vi "Combine Events.vi"(5 "NXT":T1={"Hardware"="NXT", "Flattened String"=""}) -> (1 "4134 Events":u8[](array[numeric]), 2 "NXT":T1={"Hardware"="NXT", "Flattened String"=""})   [LabVIEW 2010, in "FTC.lvlib" / "Remote Interface.lvlib"]
uses:
  Remote Interface.lvlib
  <vilib>/FTC/FTC POVState.ctl
  <vilib>/NXT/Subs/LVHSConnector.ctl
  <vilib>/NXT/Dual Mode Library/prims/dataManipulation/joinU8.vi
panel:
  in  "Old Button Encoding 2":u16
  in  "Old POV 2":T2 items=["None"=-1, "POV Up"=0, "POV Up Right"=1, "POV Right"=2, "POV Down Right"=3, "POV Down"=4, "POV Down Left"=5, "POV Left"=6, "POV Up Left"=7]
  in  "Old Button Encoding 1":u16
  in  "Old POV 1":T2 items=["None"=-1, "POV Up"=0, "POV Up Right"=1, "POV Right"=2, "POV Down Right"=3, "POV Down"=4, "POV Down Left"=5, "POV Left"=6, "POV Up Left"=7]
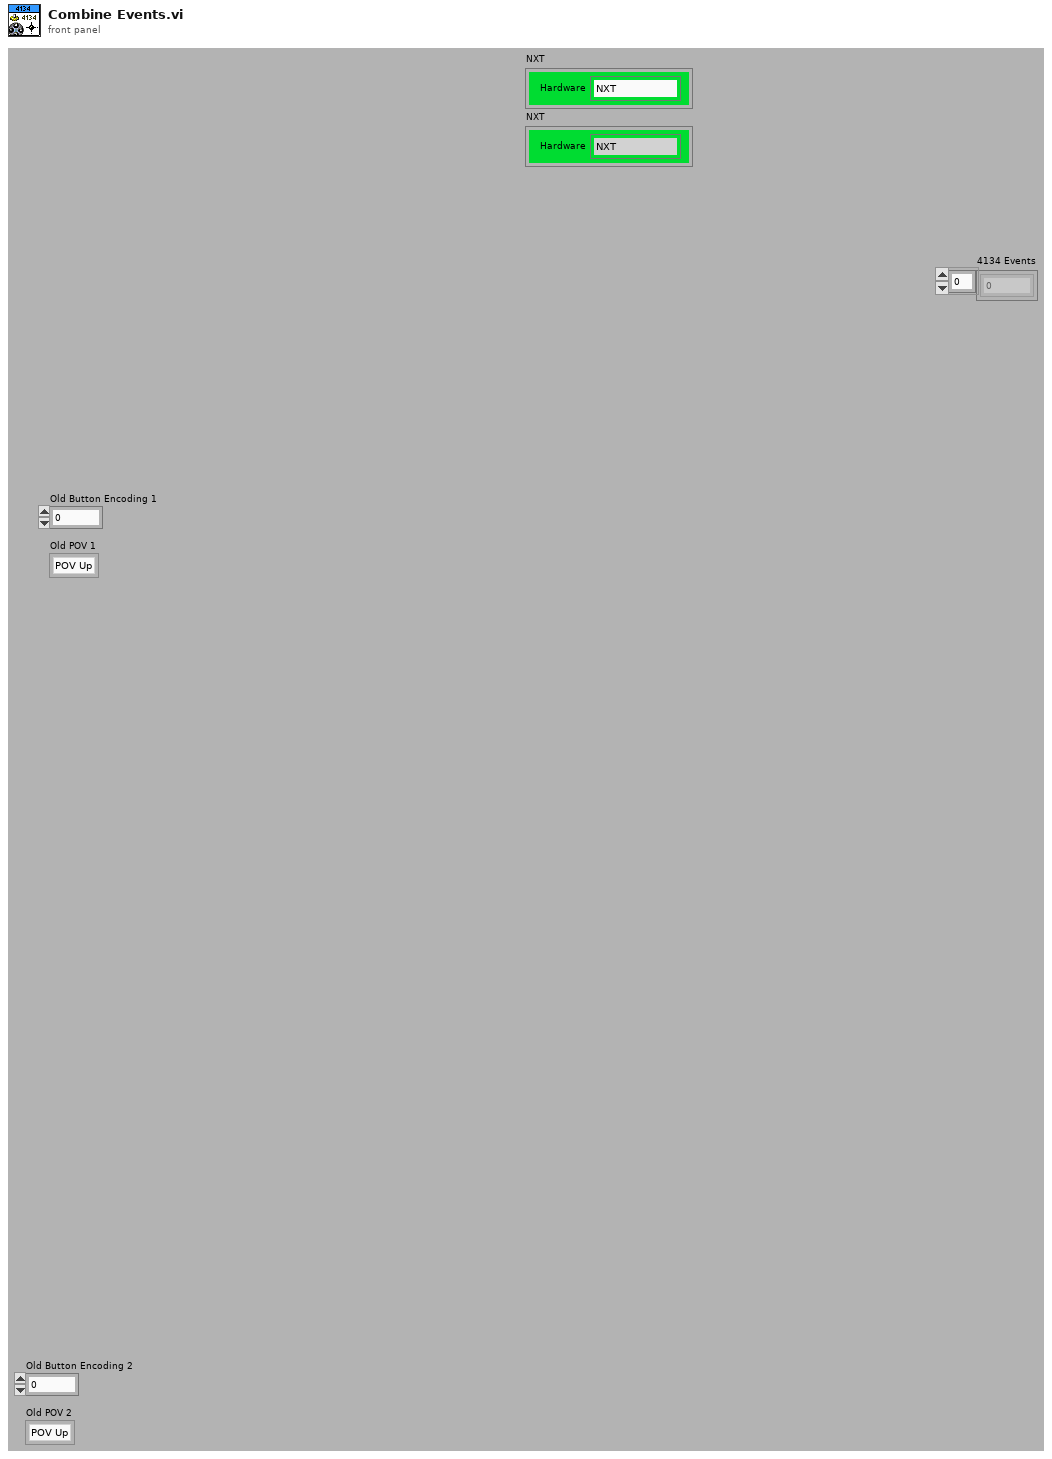
[diagram p1: front panel]
types:
  T1 = typedef "LVHSConnector.ctl" = cluster{"Hardware":string, "Flattened String":string}
  T2 = typedef "FTC POVState.ctl" = i8
  T3 = typedef "FTC ControllerState.ctl" = cluster{"Left X":i8, "Left Y":i8, "Right X":i8, "Right Y":i8, "Button Encoding 9-12":u8, "Button Encoding 1-8":u8, "POV":T2}
  T4 = enum16{"Pressed", "Released", "Toggled", "Untoggled"}
  T5 = enum16{"1-1", "1-2", "1-3", "1-4", "1-5", "1-6", "1-7", "1-8", "1-9", "1-10", "1-11", "1-12", "2-1", "2-2", "2-3", "2-4", "2-5", "2-6", "2-7", "2-8", "2-9", "2-10", "2-11", "2-12", "NXT-L", "NXT-R", "NXT-E", "1-U", "1-UR", "1-R", "1-DR", "1-D", "1-DL", "1-L", "1-UL", "2-U", "2-UR", "2-R", "2-DR", "2-D", "2-DL", "2-L", "2-UL"}
  T6 = enum8{"Pressed", "Released", "Toggled", "Untoggled"}
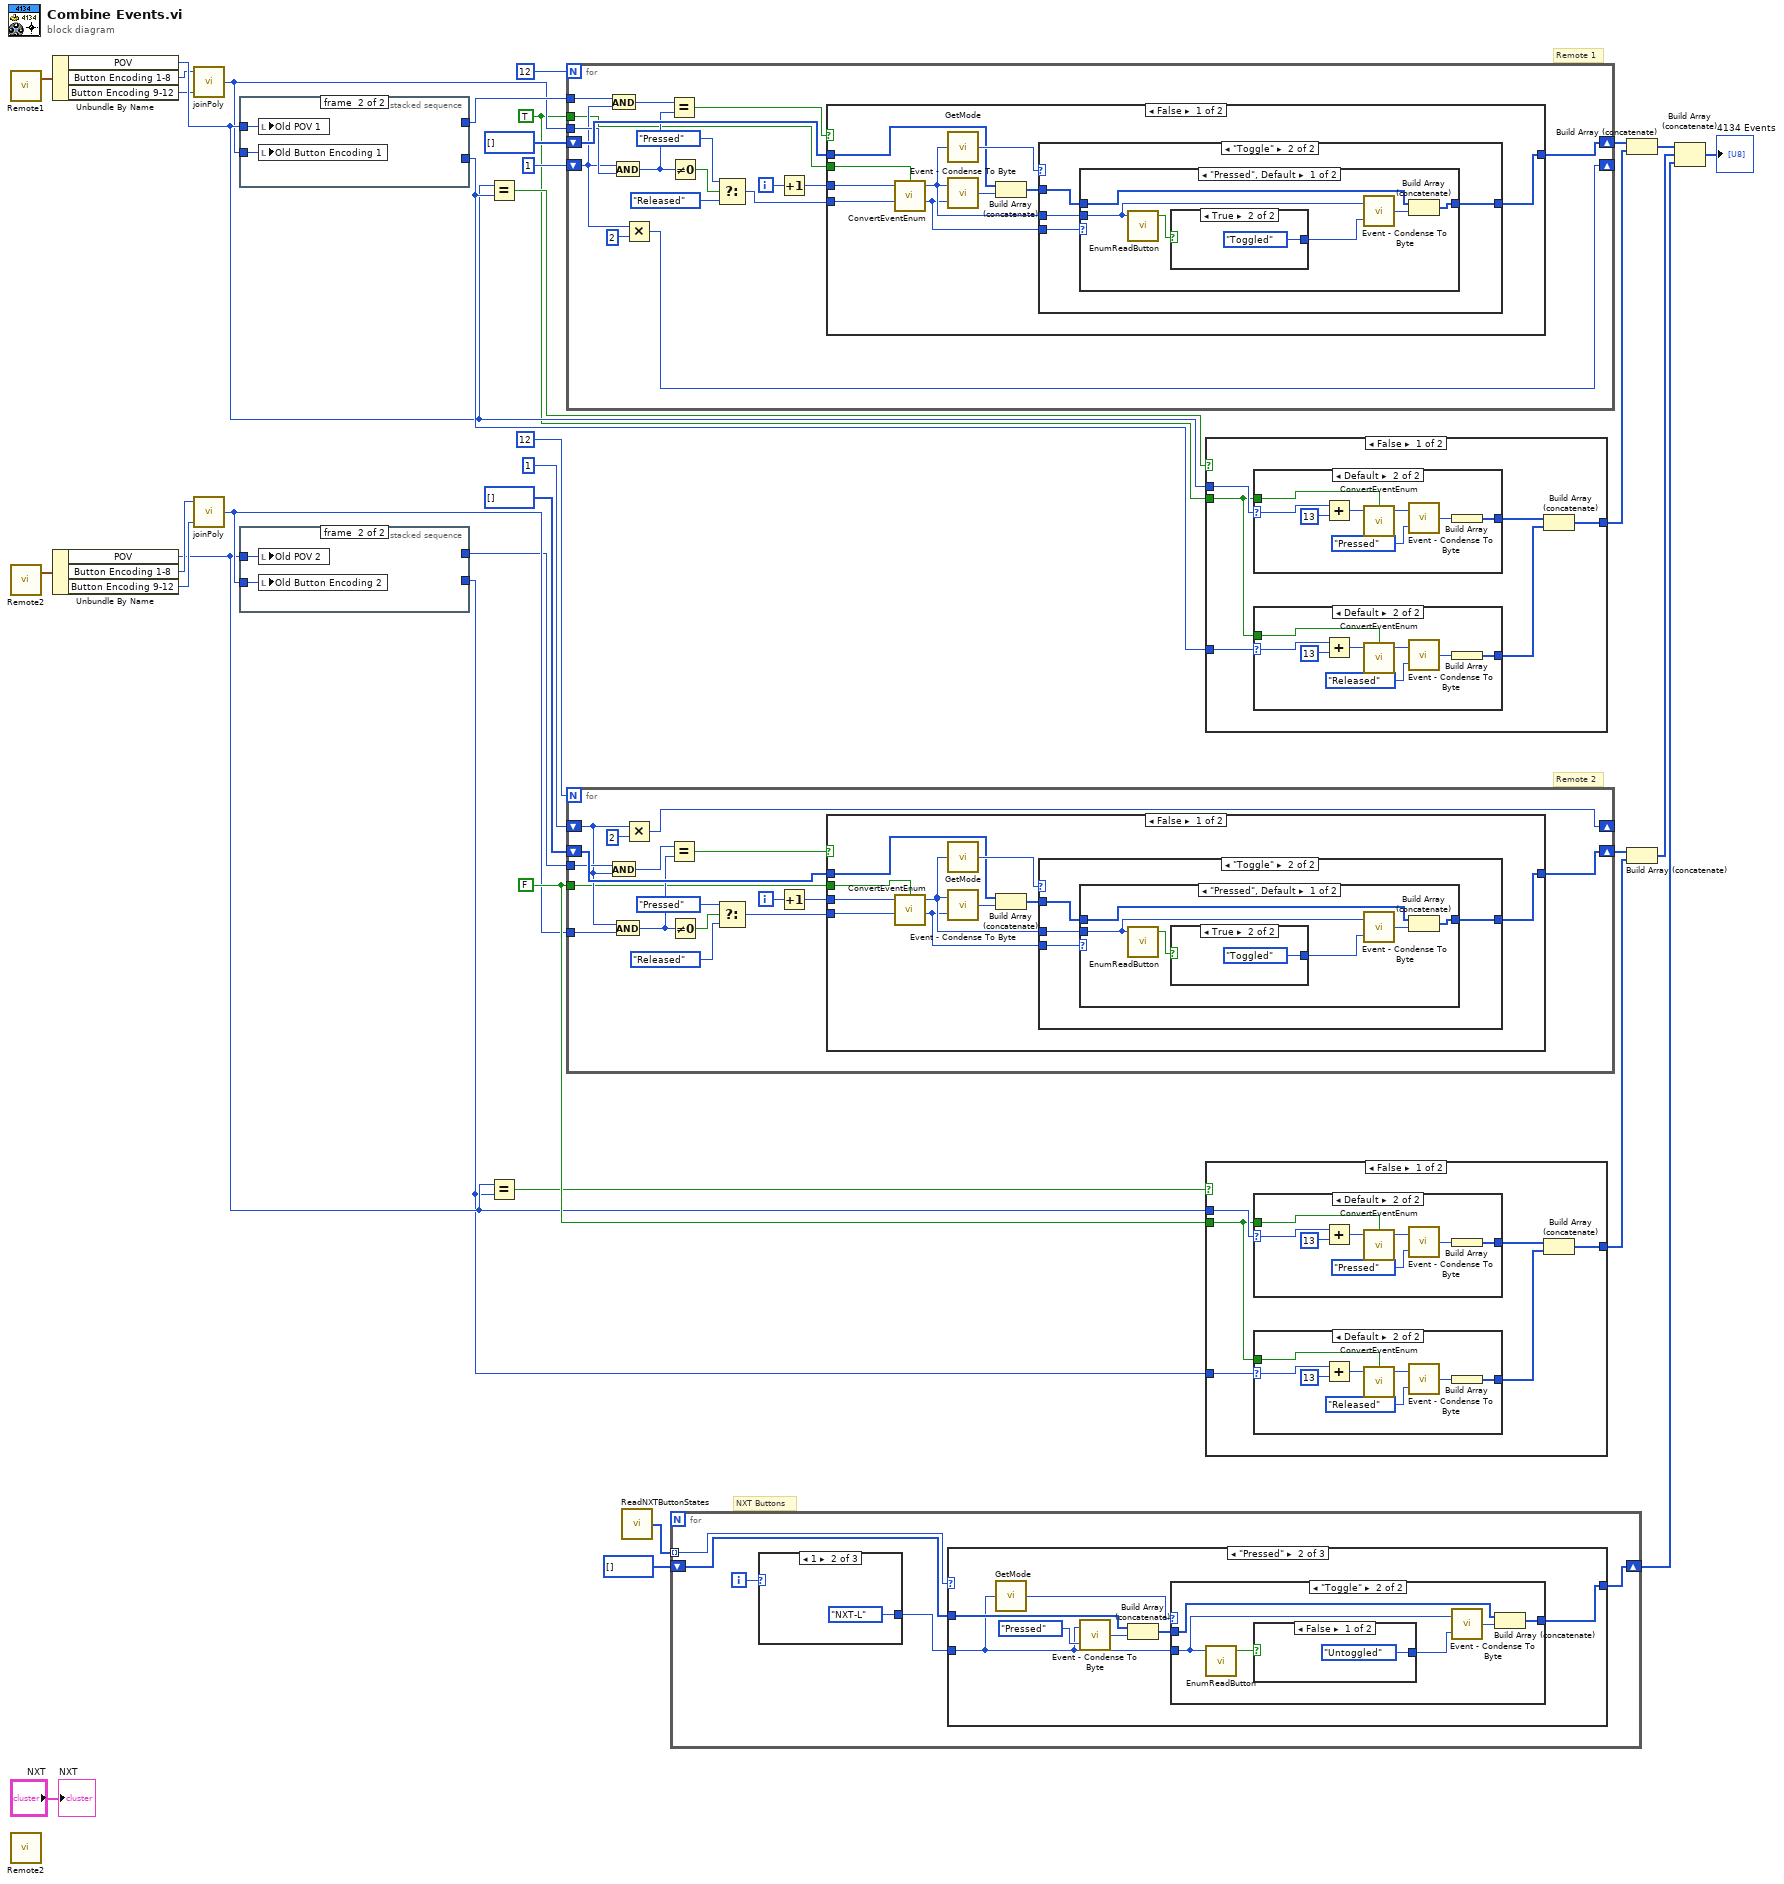
[diagram p0: block diagram]
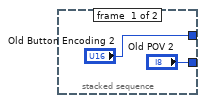
[diagram p5: hidden frame]
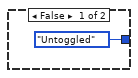
[diagram p7: hidden frame]
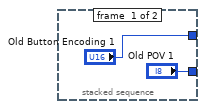
[diagram p13: hidden frame]
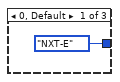
[diagram p14: hidden frame]
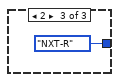
[diagram p15: hidden frame]
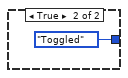
[diagram p18: hidden frame]
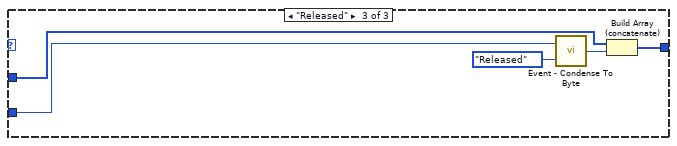
[diagram p19: hidden frame]
diagram:
  w20 = FALSE ("Crtl1?")
  w21 = TRUE ("Crtl1?")
  # "Remote 2"
  # "NXT Buttons"
  # "Remote 1"
  n1 = call "Remote1.vi"() -> ("Controller State"=w31:T3)  [unwired: 4 in]
  n2 = call "Remote2.vi"() -> ("Controller State"=w7:T3)  [unwired: 4 in]
  n3 = call "Remote2.vi"() -> ()  [unwired: 4 in, 1 out]
  n4 = Unbundle By Name(w31) -> ("POV"=w32:T2, "Button Encoding 1-8"=w30:u8, "Button Encoding 9-12"=w29:u8)
  n5 = Unbundle By Name(w7) -> ("POV"=w10:T2, "Button Encoding 1-8"=w11:u8, "Button Encoding 9-12"=w12:u8)
  n6 = call-poly <vilib>:"joinPoly.vi"("lo"=w29, "hi"=w30) -> ("(hi-lo)"=w24:u16)  [unwired: 3 in]
  n7 = call-poly <vilib>:"joinPoly.vi"("lo"=w12, "hi"=w11) -> ("(hi-lo)"=w17:u16)  [unwired: 3 in]
  n8 = stacked-sequence {
    tunnel: ["Old Button Encoding 1" _] -> w25
    tunnel: w24 -> [_ w39]
    tunnel: w32 -> [_ w38]
    tunnel: ["Old POV 1" _] -> w34
    frame #0 {
    }
    frame #1 {
      n9 = local write "Old POV 1"(w38) -> ()
      n10 = local write "Old Button Encoding 1"(w39) -> ()
    }
  }
  n11 = stacked-sequence {
    tunnel: ["Old Button Encoding 2" _] -> w16
    tunnel: w17 -> [_ w43]
    tunnel: w10 -> [_ w42]
    tunnel: ["Old POV 2" _] -> w8
    frame #0 {
    }
    frame #1 {
      n12 = local write "Old POV 2"(w42) -> ()
      n13 = local write "Old Button Encoding 2"(w43) -> ()
    }
  }
  n14 = Equal?(x=w32, y=w34) -> (x = y?=w33:bool)
  n15 = Equal?(x=w10, y=w8) -> (x = y?=w9:bool)
  n16 = for {
    N: 12 -> [_]
    shift-right: [w59] -> w28
    shift-left: u8[] [] -> [w60]
    tunnel: w25 -> [w54]
    tunnel: w24 -> [w53]
    shift-right: [w51] -> _
    shift-left: u16 1 -> [w52]
    tunnel: w21 -> [w44]
    i -> [w50]
    n17 = And(x=w54, y=w52) -> (x .and. y?=w58:u16)
    n18 = And(x=w52, y=w53) -> (x .and. y?=w57:u16)
    n19 = Multiply(x=w52, y=u16 2) -> (x*y=w51:u16)
    n20 = Equal?(x=w58, y=w57) -> (x = y?=w47:bool)
    n21 = Not Equal To 0?(x=w57) -> (x != 0?=w56:bool)
    n22 = Select(t=enum16{"Pressed", "Released"}."Pressed" ("Event Type"), s=w56, f=enum16{"Pressed", "Released"}."Released" ("Event Type")) -> (s? t:f=w45:enum16{"Pressed", "Released"})
    n23 = Increment(x=w50) -> (x+1=w46:i32)
    n24 = case shown="False" w47 {
      tunnel: w45 -> [w62 _]
      tunnel: w46 -> [w69 _]
      tunnel: w60 -> [w67 w84]
      tunnel: [w63 w84] -> w59
      tunnel: w44 -> [w61 _]
      frame False {
        n25 = call "ConvertEventEnum.vi"("Button ID"=w69, "Crtl1?"=w61) -> ("4134 Button ID"=w64:T5)  [unwired: 3 in]
        n26 = call "GetMode.vi"("Button"=w64) -> ("Mode"=w68:enum16{"Default", "Toggle"})
        n27 = call "Event - Condense To Byte.vi"("4134 Event Type"=w62, "4134 Button ID"=w64) -> ("8-bit event"=w65:u8)
        n28 = Build Array (concatenate)(w67, w65) -> (w66:u8[])
        n29 = case shown="\"Toggle\"" w68 {
          tunnel: w66 -> [w70 w72]
          tunnel: w62 -> [_ w74]
          tunnel: [w70 w73] -> w63
          tunnel: w64 -> [_ w71]
          frame "Default", Default {
          }
          frame "Toggle" {
            n30 = case shown="\"Pressed\", Default" w74 {
              tunnel: [w77 w83] -> w73
              tunnel: w72 -> [w78 w83]
              tunnel: w71 -> [w75 _]
              frame "Pressed", Default {
                n31 = call "EnumReadButton.vi"("Button"=w75) -> ("Pressed?"=w80:bool)  [unwired: 4 in]
                n32 = case shown="True" w80 {
                  tunnel: [T4."Untoggled" ("4134 Event Type") T4."Toggled" ("4134 Event Type")] -> w76
                  frame False {
                  }
                  frame True {
                  }
                }
                n33 = call "Event - Condense To Byte.vi"("4134 Event Type"=w76, "4134 Button ID"=w75) -> ("8-bit event"=w79:u8)
                n34 = Build Array (concatenate)(w78, w79) -> (w77:u8[])
              }
              frame "Released" {
              }
            }
          }
        }
      }
      frame True {
      }
    }
  }
  n35 = for {
    N: 12 -> [_]
    shift-right: [w100] -> w13
    shift-left: u8[] [] -> [w101]
    tunnel: w16 -> [w95]
    tunnel: w17 -> [w94]
    shift-right: [w92] -> _
    shift-left: u16 1 -> [w93]
    tunnel: w20 -> [w85]
    i -> [w91]
    n36 = And(x=w95, y=w93) -> (x .and. y?=w99:u16)
    n37 = And(x=w93, y=w94) -> (x .and. y?=w98:u16)
    n38 = Multiply(x=w93, y=u16 2) -> (x*y=w92:u16)
    n39 = Equal?(x=w99, y=w98) -> (x = y?=w88:bool)
    n40 = Not Equal To 0?(x=w98) -> (x != 0?=w97:bool)
    n41 = Select(t=enum16{"Pressed", "Released"}."Pressed" ("Event Type"), s=w97, f=enum16{"Pressed", "Released"}."Released" ("Event Type")) -> (s? t:f=w86:enum16{"Pressed", "Released"})
    n42 = Increment(x=w91) -> (x+1=w87:i32)
    n43 = case shown="False" w88 {
      tunnel: w86 -> [w103 _]
      tunnel: w87 -> [w110 _]
      tunnel: w101 -> [w108 w125]
      tunnel: [w104 w125] -> w100
      tunnel: w85 -> [w102 _]
      frame False {
        n44 = call "ConvertEventEnum.vi"("Button ID"=w110, "Crtl1?"=w102) -> ("4134 Button ID"=w105:T5)  [unwired: 3 in]
        n45 = call "GetMode.vi"("Button"=w105) -> ("Mode"=w109:enum16{"Default", "Toggle"})
        n46 = call "Event - Condense To Byte.vi"("4134 Event Type"=w103, "4134 Button ID"=w105) -> ("8-bit event"=w106:u8)
        n47 = Build Array (concatenate)(w108, w106) -> (w107:u8[])
        n48 = case shown="\"Toggle\"" w109 {
          tunnel: w107 -> [w111 w113]
          tunnel: w103 -> [_ w115]
          tunnel: [w111 w114] -> w104
          tunnel: w105 -> [_ w112]
          frame "Default", Default {
          }
          frame "Toggle" {
            n49 = case shown="\"Pressed\", Default" w115 {
              tunnel: [w118 w124] -> w114
              tunnel: w113 -> [w119 w124]
              tunnel: w112 -> [w116 _]
              frame "Pressed", Default {
                n50 = call "EnumReadButton.vi"("Button"=w116) -> ("Pressed?"=w121:bool)  [unwired: 4 in]
                n51 = case shown="True" w121 {
                  tunnel: [T4."Untoggled" ("4134 Event Type") T4."Toggled" ("4134 Event Type")] -> w117
                  frame False {
                  }
                  frame True {
                  }
                }
                n52 = call "Event - Condense To Byte.vi"("4134 Event Type"=w117, "4134 Button ID"=w116) -> ("8-bit event"=w120:u8)
                n53 = Build Array (concatenate)(w119, w120) -> (w118:u8[])
              }
              frame "Released" {
              }
            }
          }
        }
      }
      frame True {
      }
    }
  }
  n54 = call "ReadNXTButtonStates.vi"() -> ("3 Button Events"=w35:enum16{"None", "Pressed", "Released"}[])
  n55 = for {
    tunnel: w35 -> [w130] mode=indexing
    shift-right: [w128] -> w3
    shift-left: u8[] [] -> [w129]
    i -> [w126]
    n56 = case shown="1" w126 {
      tunnel: [T5."NXT-E" ("4134 Button ID") T5."NXT-L" ("4134 Button ID") T5."NXT-R" ("4134 Button ID")] -> w127
      frame 0, Default {
      }
      frame 1 {
      }
      frame 2 {
      }
    }
    n57 = case shown="\"Pressed\"" w130 {
      tunnel: w129 -> [w134 w138 w155]
      tunnel: [w134 w135 w153] -> w128
      tunnel: w127 -> [_ w137 w151]
      frame "None", Default {
      }
      frame "Pressed" {
        n58 = call "GetMode.vi"("Button"=w137) -> ("Mode"=w141:enum16{"Default", "Toggle"})
        n59 = call "Event - Condense To Byte.vi"("4134 Event Type"=T4."Pressed", "4134 Button ID"=w137) -> ("8-bit event"=w140:u8)
        n60 = Build Array (concatenate)(w138, w140) -> (w136:u8[])
        n61 = case shown="\"Toggle\"" w141 {
          tunnel: w137 -> [_ w144]
          tunnel: w136 -> [w142 w145]
          tunnel: [w142 w143] -> w135
          frame "Default", Default {
          }
          frame "Toggle" {
            n62 = call "EnumReadButton.vi"("Button"=w144) -> ("Pressed?"=w148:bool)  [unwired: 4 in]
            n63 = case shown="False" w148 {
              tunnel: [T4."Untoggled" ("4134 Event Type") T4."Toggled" ("4134 Event Type")] -> w146
              frame False {
              }
              frame True {
              }
            }
            n64 = call "Event - Condense To Byte.vi"("4134 Event Type"=w146, "4134 Button ID"=w144) -> ("8-bit event"=w147:u8)
            n65 = Build Array (concatenate)(w145, w147) -> (w143:u8[])
          }
        }
      }
      frame "Released" {
        n66 = call "Event - Condense To Byte.vi"("4134 Event Type"=T4."Released", "4134 Button ID"=w151) -> ("8-bit event"=w154:u8)
        n67 = Build Array (concatenate)(w155, w154) -> (w153:u8[])
      }
    }
  }
  n68 = case shown="False" w33 {
    tunnel: w34 -> [w160 _]
    tunnel: w32 -> [w161 _]
    tunnel: [w158 _] -> w27
    tunnel: w21 -> [w156 _]
    frame False {
      n69 = case shown="Default" w161 {
        selector: w161 -> [_ w176]
        tunnel: [_ w171] -> w159
        tunnel: w156 -> [_ w170]
        frame -1 {
        }
        frame Default {
          n70 = Add(x=w176, y=u16 13) -> (x+y=w175:u16)
          n71 = call "ConvertEventEnum.vi"("Button ID"=w175, "Crtl1?"=w170) -> ("4134 Button ID"=w174:T5)  [unwired: 3 in]
          n72 = call "Event - Condense To Byte.vi"("4134 Event Type"=T6."Pressed", "4134 Button ID"=w174) -> ("8-bit event"=w172:u8)
          n73 = Build Array(w172) -> (w171:u8[])
        }
      }
      n74 = case shown="Default" w160 {
        selector: w160 -> [_ w169]
        tunnel: [_ w164] -> w157
        tunnel: w156 -> [_ w162]
        frame -1 {
        }
        frame Default {
          n75 = Add(x=w169, y=u16 13) -> (x+y=w167:u16)
          n76 = call "ConvertEventEnum.vi"("Button ID"=w167, "Crtl1?"=w162) -> ("4134 Button ID"=w166:T5)  [unwired: 3 in]
          n77 = call "Event - Condense To Byte.vi"("4134 Event Type"=T6."Released", "4134 Button ID"=w166) -> ("8-bit event"=w163:u8)
          n78 = Build Array(w163) -> (w164:u8[])
        }
      }
      n79 = Build Array (concatenate)(w159, w157) -> (w158:u8[])
    }
    frame True {
    }
  }
  n80 = case shown="False" w9 {
    tunnel: w8 -> [w182 _]
    tunnel: w10 -> [w183 _]
    tunnel: [w180 _] -> w14
    tunnel: w20 -> [w178 _]
    frame False {
      n81 = case shown="Default" w183 {
        selector: w183 -> [_ w198]
        tunnel: [_ w193] -> w181
        tunnel: w178 -> [_ w192]
        frame -1 {
        }
        frame Default {
          n82 = Add(x=w198, y=u16 13) -> (x+y=w197:u16)
          n83 = call "ConvertEventEnum.vi"("Button ID"=w197, "Crtl1?"=w192) -> ("4134 Button ID"=w196:T5)  [unwired: 3 in]
          n84 = call "Event - Condense To Byte.vi"("4134 Event Type"=T6."Pressed", "4134 Button ID"=w196) -> ("8-bit event"=w194:u8)
          n85 = Build Array(w194) -> (w193:u8[])
        }
      }
      n86 = case shown="Default" w182 {
        selector: w182 -> [_ w191]
        tunnel: [_ w186] -> w179
        tunnel: w178 -> [_ w184]
        frame -1 {
        }
        frame Default {
          n87 = Add(x=w191, y=u16 13) -> (x+y=w189:u16)
          n88 = call "ConvertEventEnum.vi"("Button ID"=w189, "Crtl1?"=w184) -> ("4134 Button ID"=w188:T5)  [unwired: 3 in]
          n89 = call "Event - Condense To Byte.vi"("4134 Event Type"=T6."Released", "4134 Button ID"=w188) -> ("8-bit event"=w185:u8)
          n90 = Build Array(w185) -> (w186:u8[])
        }
      }
      n91 = Build Array (concatenate)(w181, w179) -> (w180:u8[])
    }
    frame True {
    }
  }
  n92 = Build Array (concatenate)(w28, w27) -> (w5:u8[])
  n93 = Build Array (concatenate)(w13, w14) -> (w4:u8[])
  n94 = Build Array (concatenate)(w5, w4, w3) -> (→"4134 Events":u8[])
  "NXT" <- "NXT"
